vi "Get Color.vi"(8 "error in (no error)":errorcluster, 11 "object in":refnum<class "Game Component.lvclass">) -> (0 "error out":errorcluster, 2 "Color":u32, 3 "object out":refnum<class "Game Component.lvclass">)   [LabVIEW 2017, in "Game Component.lvclass"]
uses:
  Game Component.lvclass
  Game Component.lvclass/Game Component.ctl
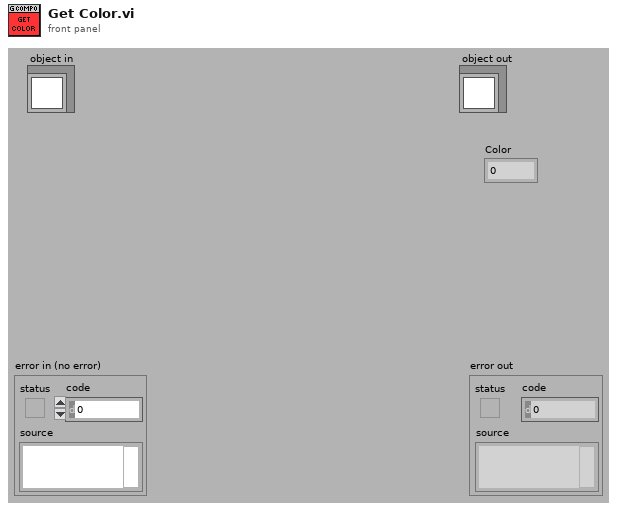
[diagram p1: front panel]
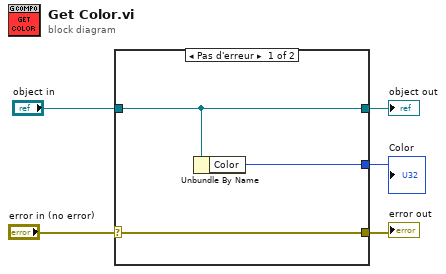
[diagram p0: block diagram]
diagram:
  n1 = case shown="Pas d'erreur" "error in (no error)" {
    selector: "error in (no error)" -> [w7 w10]
    tunnel: [w7 w10] -> w4
    tunnel: [w6 w9] -> w2
    tunnel: "object in" -> [w6 w9]
    tunnel: [w8 _] -> w1
    frame No Error {
      n2 = Unbundle By Name(w6) -> ("Color"=w8:u32)
    }
    frame Error {
    }
  }
  "error out" <- w4
  "object out" <- w2
  "Color" <- w1
